vi "Write Build Data.vi"(0 "Build Named Build Specification Data in":refnum<class "Build Named Build Specification Data.lvclass">, 5 "Generated files":path[](array[path]), 7 "Build Specification Name":string, 9 "Target Name":string, 11 "error in (no error)":errorcluster) -> (4 "Build Named Build Specification Data out":refnum<class "Build Named Build Specification Data.lvclass">, 15 "error out":errorcluster)   [LabVIEW 2019, in "ProjectBuilder.lvlib" / "Build Named Build Specification Data.lvclass"]
doc: "Write private data."
uses:
  Build Named Build Specification Data.lvclass
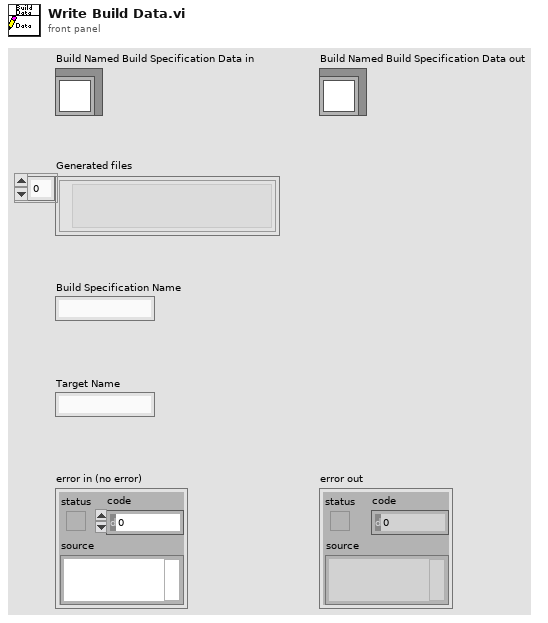
[diagram p1: front panel]
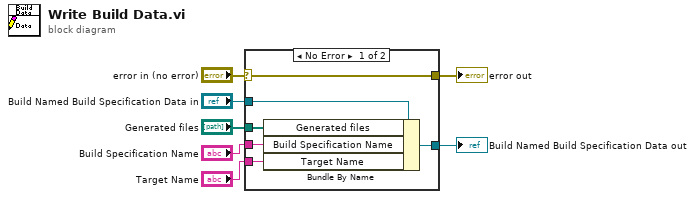
[diagram p0: block diagram]
diagram:
  n1 = case shown="No Error" "error in (no error)" {
    selector: "error in (no error)" -> [w13 w14]
    tunnel: [w13 w14] -> w6
    tunnel: [w11 w15] -> w4
    tunnel: "Build Named Build Specification Data in" -> [w12 w15]
    tunnel: "Generated files" -> [w10 _]
    tunnel: "Build Specification Name" -> [w9 _]
    tunnel: "Target Name" -> [w8 _]
    frame No Error {
      n2 = Bundle By Name(cluster=w12, "Generated files"=w10, "Build Specification Name"=w9, "Target Name"=w8) -> (w11:refnum<class "Build Named Build Specification Data.lvclass">)
    }
    frame Error {
    }
  }
  "error out" <- w6
  "Build Named Build Specification Data out" <- w4
